vi "Set Multi Gate Inverted [GIN].vi"(6 "Gate Number":i32, 7 "Micropulse # In":i32, 8 "error in (no error)":errorcluster, 9 "Inverted?":bool, 11 "Test Number":u32) -> (0 "error out":errorcluster, 5 "Micropulse # Out":i32)   [LabVIEW 2026, in "MicroPulse_Driver.lvlib"]
doc: "To allow the detection of negative peaks in a gate. This function is intended for use with RF signals and the UML value now becomes the threshold for reporting when the signal breaks it in a negative direction\n\nParameters:\n<Tn> : Test number. An integer value from 0 to the maximum number of tests (default maximum is 1279 tests).\nTn = 0 for all conventional tests. If the S extension is used it applies to all tests in the sweep number specified: 1-32, 0 = all sweeps.\n\n<Gn> : Gate Number, an integer value from 0 to 4.\nGn = 0 for all gates in the test\n\n<value> : Integer 0 between 1\n0 = normal positive peak detection gate\n1 = negative peak detection gate\n\nExample:\nDOF 1\nGAT 1 0 5000\nAMP 1 32\nAWF 1 1\nGMT 1 1 1000 4000\nGML 1 2 1000 4000\nGIN 1 2 1\nAMM 1 0 1\nUML 1 1 154\nUML 1 2 100\n\nIn this example gates 1 and 2 are looking at RF data in 8-bit mode (normally 127). In gate 1 the largest positive going signal that breaks the 154 threshold will be reported, while in gate 2 the largest negative going signal that breaks the 100 threshold will be reported.\n\nNote:\nValid in Multi-gate Mode only (AMP 31 & 32)\n<b>To ensure the correct threshold is set for a gate the UML command should be re-sent after the GIN command.</b>"
uses:
  MicroPulse_Driver.lvlib
  Private/MP-Registry Action-Enum.ctl
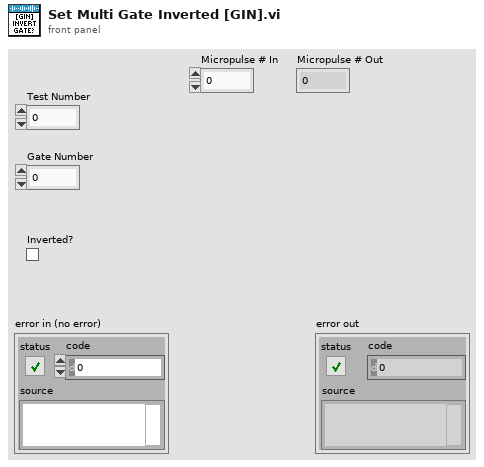
[diagram p1: front panel]
types:
  T1 = typedef "MicroPulse_Driver.lvlib/MP-Registry Action-Enum.ctl" = enum16{"Read", "Add Test", "Add Command", "Add Gate Command", "Add Encoder Command", "Clear Command  List", "Set Registry", "Set System Details", "Set DOF", "Set Velocity", "Disable Asynch Reads", "Enable Asynch Reads", "Add Connection", "Disconnect", "Shutdown"}
  T2 = typedef "Micropulse.lvlib/TCP config.ctl" = cluster{"Connection ID":refnum<k5>, "IP address":string, "host port":u16, "OC timeout":i32, "Read timeout":i32, "Write timeout":i32}
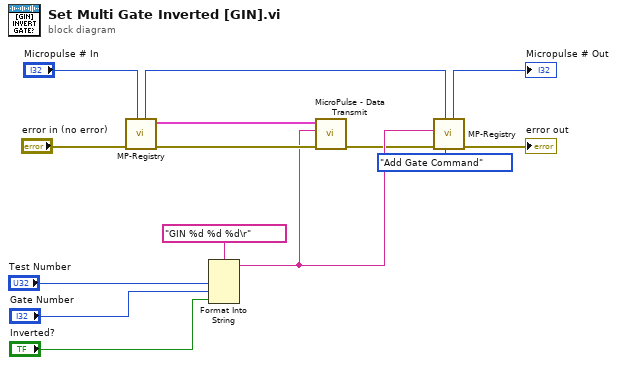
[diagram p0: block diagram]
diagram:
  n1 = call "MP-Registry.vi"("Micropulse # In"="Micropulse # In", "error in (no error)"="error in (no error)") -> ("error out"=w12:errorcluster, "TCP config"=w11:T2, "Micropulse # Out"=w5:i32)  [unwired: 6 in, 1 out]
  n2 = Format Into String(format string="GIN %d %d %d\r", "Test Number", "Gate Number", "Inverted?") -> (resulting string=w9:string)  [unwired: 2 in, 1 out]
  n3 = call "MicroPulse - Data Transmit.vi"("error in (no error)"=w12, "data"=w9, "TCP config"=w11) -> ("error out"=w7:errorcluster)  [unwired: 6 in, 2 out]
  n4 = call "MP-Registry.vi"("Action"=MP-Registry_Action-Enum."Add Gate Command", "Micropulse # In"=w5, "error in (no error)"=w7, "Data in"=w9) -> ("error out"=→"error out":errorcluster, "Micropulse # Out"=→"Micropulse # Out":i32)  [unwired: 4 in, 2 out]
